vi "DeepClone.vi"(8 "error in (no error)":errorcluster, 11 "Object (subject) in":refnum<class "Object (subject).lvclass">) -> (0 "error out":errorcluster, 2 "Copy":refnum<class "Object (subject).lvclass">, 3 "Object (subject) out":refnum<class "Object (subject).lvclass">)   [LabVIEW 2014, in "Object (subject).lvclass"]
uses:
  Object (subject).lvclass
  Object (subject).lvclass/Object (subject).ctl
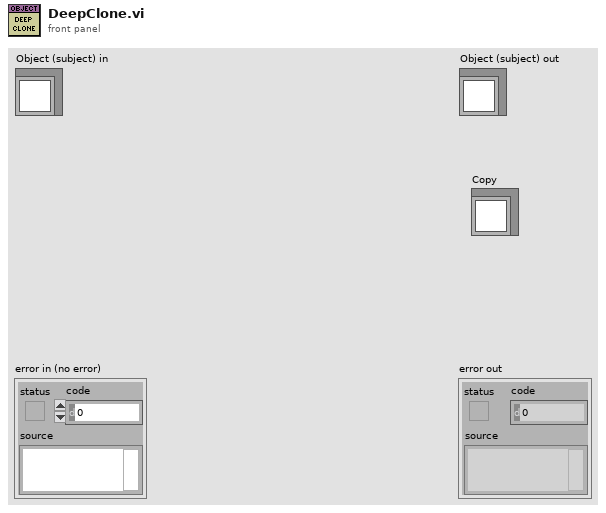
[diagram p1: front panel]
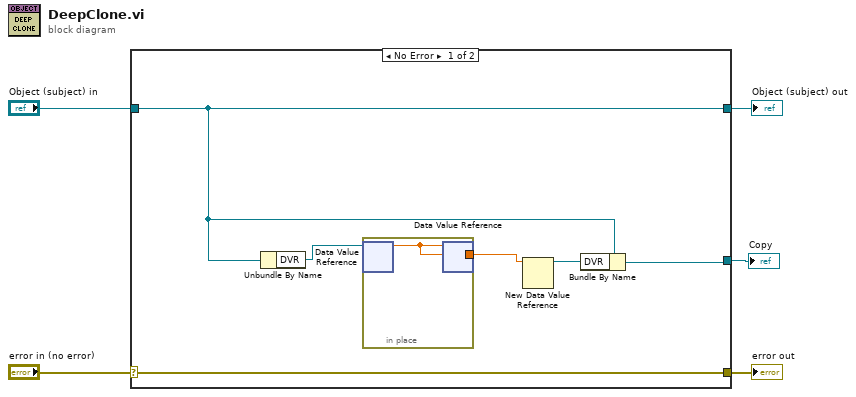
[diagram p0: block diagram]
diagram:
  n1 = case shown="No Error" "error in (no error)" {
    selector: "error in (no error)" -> [w11 w14]
    tunnel: [w11 w14] -> w4
    tunnel: [w10 w13] -> w2
    tunnel: "Object (subject) in" -> [w10 w13]
    tunnel: [w8 _] -> w1
    frame No Error {
      n2 = Unbundle By Name(w10) -> ("DVR"=w7:refnum<data-value>)
      n3 = in-place {
        in-place-border: [w12] -> w6
        n4 = in-place-dvr #1(w7) -> (w12:dbl)  [unwired: 1 out]
        n5 = in-place-dvr #1(w12) -> ()  [unwired: 2 out]
      }
      n6 = New Data Value Reference(data value=w6) -> (data value reference=w9:refnum<data-value>)  [unwired: 1 in, 1 out]
      n7 = Bundle By Name(cluster=w10, "DVR"=w9) -> (w8:refnum<class "Object (subject).lvclass">)
    }
    frame Error {
    }
  }
  "error out" <- w4
  "Object (subject) out" <- w2
  "Copy" <- w1
